vi "ConnectToCamera.vi"() -> (2 "Camera data (out)":variant, 3 "Camera interface":T1)   [LabVIEW 2011]
uses:
  CameraInterface/CameraInterface.ctl
  CameraInterface/CICloseType.ctl
  CameraInterface/CIGetSetGenericConfig.ctl
  CameraInterface/CIGrabType.ctl
  CameraInterface/CISettingsDlg.ctl
  CameraInterface/CIAdjustBeadPos.ctl
  CameraInterface/CISaveLoadSettings.ctl
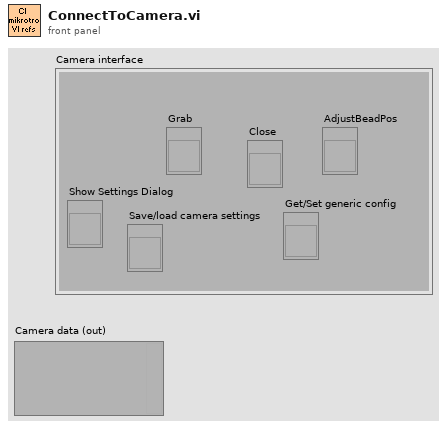
[diagram p1: front panel]
types:
  T1 = typedef "CameraInterface.ctl" = cluster{"Close":T2, "Get/Set generic config":T3, "Grab":T4, "Show Settings Dialog":T5, "AdjustBeadPos":T6, "Save/load camera settings":T7}
  T2 = typedef "CICloseType.ctl" = refnum<vi>
  T3 = typedef "CIGetSetGenericConfig.ctl" = refnum<vi>
  T4 = typedef "CIGrabType.ctl" = refnum<vi>
  T5 = typedef "CISettingsDlg.ctl" = refnum<vi>
  T6 = typedef "CIAdjustBeadPos.ctl" = refnum<vi>
  T7 = typedef "CISaveLoadSettings.ctl" = refnum<vi>
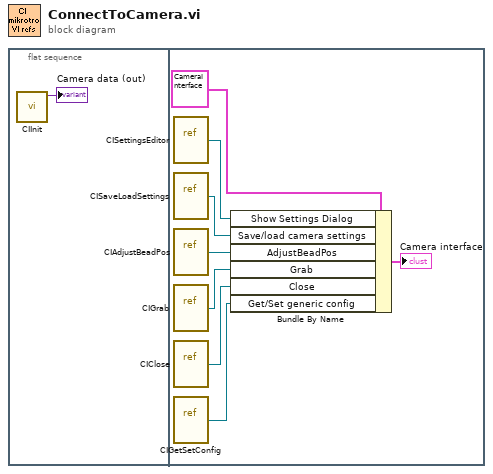
[diagram p0: block diagram]
diagram:
  n1 = flat-sequence {
    frame #0 {
      n2 = call "CIInit.vi"() -> ("Camera data (out)"=→"Camera data (out)":variant)  [unwired: 11 in]
    }
    frame #1 {
      n3 = vi-ref "CISettingsEditor.vi"() -> (w8:refnum<vi>)
      n4 = vi-ref "CISaveLoadSettings.vi"() -> (w3:refnum<vi>)
      n5 = vi-ref "CIAdjustBeadPos.vi"() -> (w4:refnum<vi>)
      n6 = vi-ref "CIGrab.vi"() -> (w2:refnum<vi>)
      n7 = vi-ref "CIClose.vi"() -> (w7:refnum<vi>)
      n8 = vi-ref "CIGetSetConfig.vi"() -> (w9:refnum<vi>)
      n9 = Bundle By Name(cluster=T1 {"Close"=refnum, "Get/Set generic config"=refnum, "Grab"=refnum, "Show Settings Dialog"=refnum, "AdjustBeadPos"=refnum, "Save/load camera settings"=refnum} ("Camera interface"), "Show Settings Dialog"=w8, "Save/load camera settings"=w3, "AdjustBeadPos"=w4, "Grab"=w2, "Close"=w7, "Get/Set generic config"=w9) -> (→"Camera interface":T1)
    }
  }
